vi "1D Rectangular To Polar.vi"(1 "X":dbl[](array[numeric]) format="%0.2f", 4 "Y":dbl[](array[numeric]) format="%0.2f") -> (0 "Magnitude":dbl[](array[numeric]) format="%0.2f", 2 "Phase":dbl[](array[numeric]) format="%0.2f", 3 "error":i32)   [LabVIEW 2020, in "NI_AALPro.lvlib"]
doc: "LabVIEW no longer supports this VI. Use the Re/Im To Polar function instead.\nThis VI converts two arrays of rectangular coordinates into two arrays of polar coordinates.\nThis VI converts the arrays of rectangular coordinates into arrays of polar coordinates using the following equations:\n<b>Magnitude</b> = sqrt(<b>X</b>^2 + <b>Y</b>^2)\n<b>Phase</b> = (tan^-1)(<b>Y</b>/<b>X</b>)"
uses:
  <vilib>/Analysis/NI_AALPro.lvlib
  <resource>/lvanlys.dll
panel:
  # "1D Rectangular To Polar"
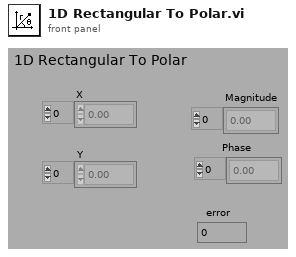
[diagram p1: front panel]
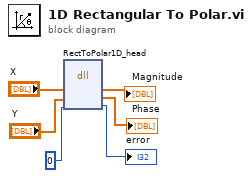
[diagram p0: block diagram]
diagram:
  n1 = dll-call lib="e:/builds/penguin/labview/branches/2020/dev/dist/resource/lvanlys.*" fn="RectToPolar1D_head"("X"="X", "Y"="Y", 0) -> ("X"=→"Magnitude":dbl[], "Y"=→"Phase":dbl[], →"error":i32)  [unwired: 4 in, 2 out]
